vi "Request Data.vi"(6 "Qualifier":string, 8 "error in":errorcluster, 9 "notifier":refnum<notifier>, 10 "Data to Send":string, 11 "DAQ970 in":refnum<class "DAQ970.lvclass">) -> (0 "error out":errorcluster, 3 "DAQ970 out":refnum<class "DAQ970.lvclass">)   [LabVIEW 2019, in "DAQ970.lvlib" / "DAQ970.lvclass"]
doc: "Data to Send is a required input that describes the measurement or query function to be performed\nQualifier is a secondary variable used in the event that specificity must be provided to the query function\n****Note****\nIf further specificity is required, the qualifier must be used in a comma delimited format to increase the overall variable count. Additional specificity must be provided by the child class and interpreted by the automated call.\n\nnotifier is a single variant notifier in which the instrument will send the data notification to the automated tool."
uses:
  Library/DAQ970.lvclass
  C:/Users/Public/Documents/Development/builds/Instruments/Instruments.lvlibp/Library/Instruments.lvclass
  builds/Instruments/Instruments.lvlibp/Accessors/Read Measured.vi
  builds/Instruments/Instruments.lvlibp/Private/Accessors/Read Poll(ms).vi
  builds/Instruments/Instruments.lvlibp/Private/Polymorphic/Special/Event from String.vi
  builds/Instruments/Instruments.lvlibp/Accessors/Command with Logging.vi
  builds/Instruments/Instruments.lvlibp/Library/Instruments.lvclass
  builds/Instruments/Instruments.lvlibp
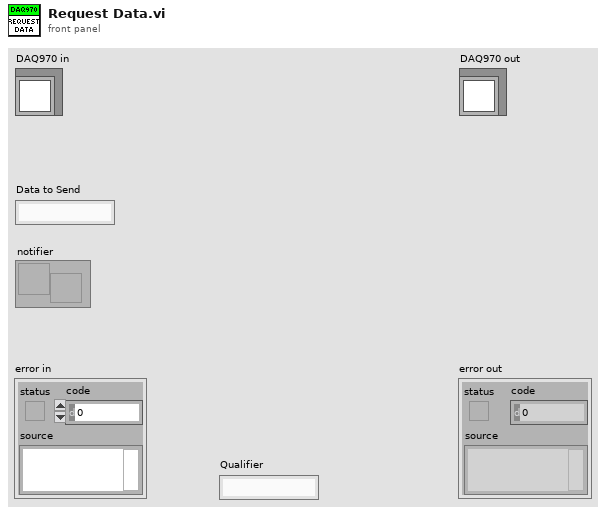
[diagram p1: front panel]
types:
  T1 = cluster{"Timestamp":timestamp, "Description":string, "Data":string}
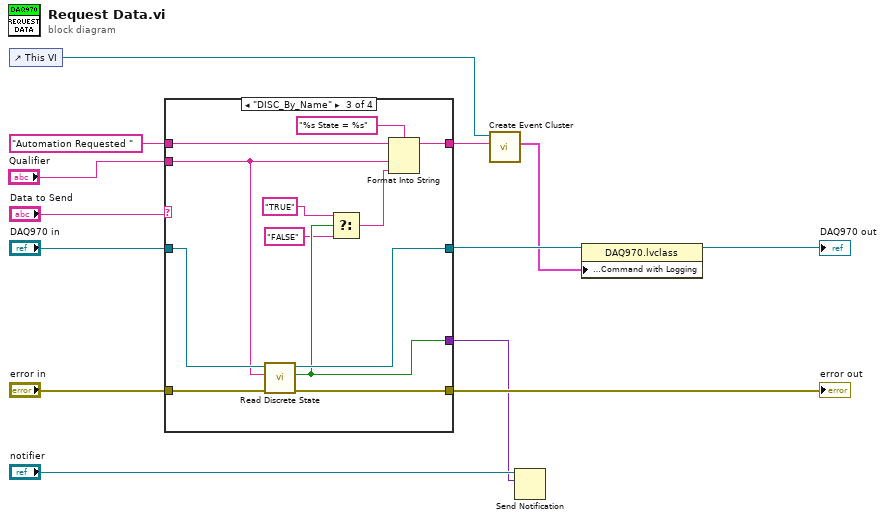
[diagram p0: block diagram]
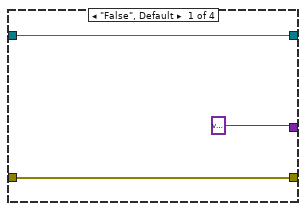
[diagram p2: hidden frame]
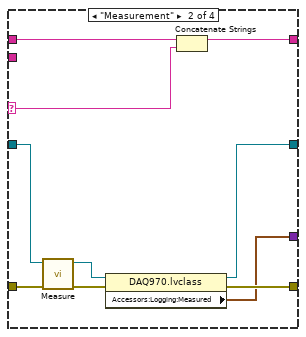
[diagram p3: hidden frame]
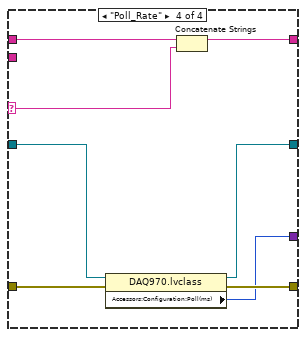
[diagram p4: hidden frame]
diagram:
  n1 = control-ref of="This VI"() -> (w13:refnum<vi>)
  n2 = case shown="\"DISC_By_Name\"" "Data to Send" {
    selector: "Data to Send" -> [_ w18 _ w40]
    tunnel: "DAQ970 in" -> [w16 w26 w34 w46]
    tunnel: "Automation Requested " -> [_ w19 w38 w41]
    tunnel: [w16 w23 w33 w45] -> w9
    tunnel: "error in" -> [w15 w21 w35 w43]
    tunnel: [w15 w22 w32 w44] -> w5
    tunnel: [variant ("Variant") w20 w30 w42] -> w3
    tunnel: [_ w17 w37 w39] -> w2
    tunnel: "Qualifier" -> [_ _ w31 _]
    frame "False", Default {
    }
    frame "Measurement" {
      n3 = call-dynamic "Measure.vi"("error in"=w21, "DAQ970 in"=w26) -> ("error out"=w25:errorcluster, "DAQ970 out"=w24:refnum<class "DAQ970.lvclass">)  [unwired: 8 in]
      n4 = property class="DAQ970.lvclass"(reference=w24, error in=w25) -> (reference out=w23:refnum<class "DAQ970.lvclass">, error out=w22:errorcluster, "Accessors:Logging:Measured"=w20:waveform(dbl)[])
      n5 = Concatenate Strings(w19, w18) -> (w17:string)
    }
    frame "DISC_By_Name" {
      n6 = call "Read Discrete State.vi"("error in"=w35, "Channel Name"=w31, "DAQ970 in"=w34) -> ("error out"=w32:errorcluster, "State"=w30:bool, "DAQ970 out"=w33:refnum<class "DAQ970.lvclass">)  [unwired: 6 in]
      n7 = Select(t="TRUE", s=w30, f="FALSE") -> (s? t:f=w27:string)
      n8 = Format Into String(format string="%s State = %s", initial string=w38, w31, w27) -> (resulting string=w37:string)  [unwired: 1 in, 1 out]
    }
    frame "Poll_Rate" {
      n9 = property class="DAQ970.lvclass"(reference=w46, error in=w43) -> (reference out=w45:refnum<class "DAQ970.lvclass">, error out=w44:errorcluster, "Accessors:Configuration:Poll(ms)"=w42:u32)
      n10 = Concatenate Strings(w41, w40) -> (w39:string)
    }
  }
  "error out" <- w5
  n11 = call-poly "Create Event Cluster.vi"("Value"=w2, "VI Refnum"=w13) -> ("Event Data"=w8:T1)  [unwired: 9 in]
  n12 = Send Notification(notification=w3, notifier="notifier") -> ()  [unwired: 1 in, 2 out]
  n13 = property class="DAQ970.lvclass"(reference=w9, "Accessors:Logging:Command with Logging"=w8) -> (reference out=→"DAQ970 out":refnum<class "DAQ970.lvclass">)  [unwired: 1 in, 1 out]
